vi "RSZVB Set Virtual Transform Ground Loop Circuit Model.vi"(7 "Circuit Model (1)":i32(ring)=1 items=["File import, no circuit model ", "Shunt L", "Shunt C"], 8 "error in (no error)":errorcluster {"code" format="%.0x"}, 9 "Function Type (0)":i32(ring) items=["Deembedding", "Embedding"], 10 "Channel (1)":i32=1, 11 "VISA session":refnum<visa-resource-name>) -> (0 "error out":errorcluster {"code" format="%.0x"}, 3 "dup VISA session":refnum<visa-resource-name>)   [LabVIEW 2011]
doc: "This VI selects the circuit model for ground loop deembedding/embedding.\n\nRemote-control command(s):\nCALCulate<Ch>:TRANsform:VNETworks:GLOop:DEEMbedding:TNDefinition FIMPort | SL | SC \nCALCulate<Ch>:TRANsform:VNETworks:GLOop:EMBedding:TNDefinition FIMPort | SL | SC"
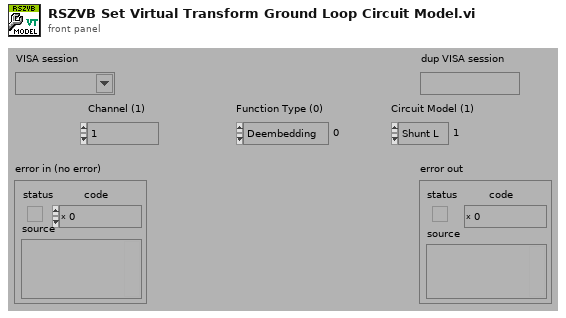
[diagram p1: front panel]
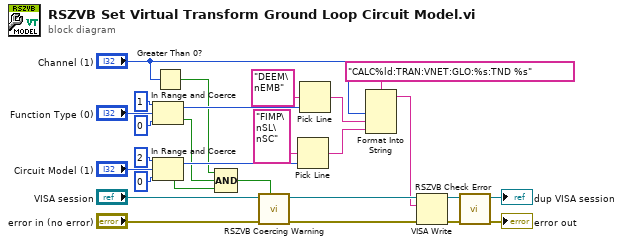
[diagram p0: block diagram]
diagram:
  n1 = In Range and Coerce(upper limit=1, x="Function Type (0)", lower limit=0) -> (coerced(x)=w14:i32, In Range?=w7:bool)
  n2 = In Range and Coerce(upper limit=2, x="Circuit Model (1)", lower limit=0) -> (coerced(x)=w9:i32, In Range?=w8:bool)
  n3 = Greater Than 0?(x="Channel (1)") -> (x > 0?=w5:bool)
  n4 = Compound Arithmetic op=AND(w5, w7, w8) -> (w4:bool)
  n5 = call "RSZVB Coercing Warning.vi"("In Range?"=w4, "error in (no error)"="error in (no error)", "VISA session"="VISA session") -> ("error out"=w23:errorcluster, "dup VISA session"=w24:refnum<visa-resource-name>)  [unwired: 7 in]
  n6 = Pick Line(multi-line string="FIMP\nSL\nSC", line index=w9) -> (output string=w3:string)  [unwired: 1 in]
  n7 = Pick Line(multi-line string="DEEM\nEMB", line index=w14) -> (output string=w18:string)  [unwired: 1 in]
  n8 = Format Into String(format string="CALC%ld:TRAN:VNET:GLO:%s:TND %s", "Channel (1)", w18, w3) -> (resulting string=w22:string)  [unwired: 2 in, 1 out]
  n9 = VISA Write(VISA resource name=w24, write buffer=w22, error in (no error)=w23) -> (VISA resource name out=w27:refnum<visa-resource-name>, error out=w26:errorcluster)  [unwired: 1 out]
  n10 = call "RSZVB Check Error.vi"("error in (no error)"=w26, "VISA session"=w27) -> ("error out"=→"error out":errorcluster, "dup VISA session"=→"dup VISA session":refnum<visa-resource-name>)  [unwired: 8 in]
